vi "Complete Call on Error.vi"(8 "error in":errorcluster, 11 "gRPC ID in":T1) -> (0 "error out":errorcluster)   [LabVIEW 2021, in "NI Measurement Plug-In SDK.lvlib" / "IMeasurement Service.lvclass"]
uses:
  IMeasurement Service.lvclass
  <vilib>/gRPC/LabVIEW gRPC Library/Shared/grpcId.ctl
  <vilib>/gRPC/LabVIEW gRPC Library/Server API/typeDefs/gRPC Status Code.ctl
  <vilib>/Utility/error.llb/DialogType.ctl
  <vilib>/gRPC/LabVIEW gRPC Library/grpc-lvsupport-release.lvlib
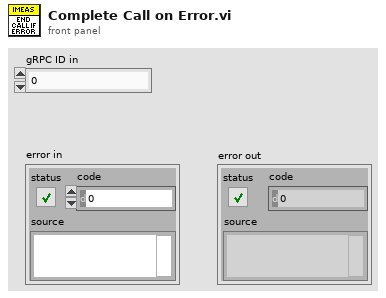
[diagram p1: front panel]
types:
  T1 = typedef "grpc-lvsupport-release.lvlib/grpcId.ctl" = u64
  T2 = typedef "grpc-lvsupport-release.lvlib/gRPC Status Code.ctl" = enum16{"OK", "CANCELLED", "UNKNOWN", "INVALID_ARGUMENT", "DEADLINE_EXCEEDED", "NOT_FOUND", "ALREADY_EXISTS", "PERMISSION_DENIED", "RESOURCE_EXHAUSTED", "FAILED_PRECONDITION", "ABORTED", "OUT_OF_RANGE", "UNIMPLEMENTED", "INTERNAL", "UNAVAILABLE", "DATA_LOSS", "UNAUTHENTICATED"}
  T3 = typedef "DialogType.ctl" = u16
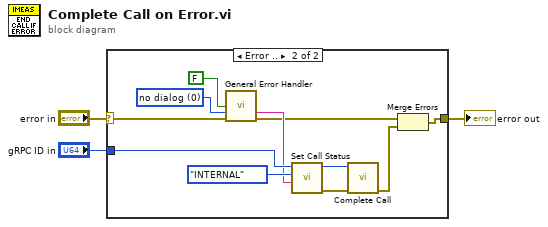
[diagram p0: block diagram]
diagram:
  n1 = case shown="Error .." "error in" {
    selector: "error in" -> [w4 w13]
    tunnel: [w4 w5] -> w1
    tunnel: "gRPC ID in" -> [_ w14]
    frame No Error {
      # "no error: pass through"
    }
    frame Error {
      w11 = T3 0 items=["no dialog", "OK message", "continue or stop message", "OK message + warnings", "continue/stop + warnings"] ("type of dialog (OK msg:1)")
      # "Report any errors over the grpc response."
      n2 = call <vilib>:"General Error Handler.vi"("search ni.com link visible?(T)"=FALSE, "type of dialog (OK msg:1)"=w11, "error in (no error)"=w13) -> ("message"=w12:string, "error out"=w6:errorcluster)  [unwired: 8 in, 3 out]
      n3 = call <vilib>:"Set Call Status.vi"("Details"=w12, "Status Code"=gRPC_Status_Code."INTERNAL", "gRPCid in"=w14) -> ("error out"=w9:errorcluster, "gRPCid out"=w8:T1)  [unwired: 7 in]
      n4 = call <vilib>:"Complete Call.vi"("gRPCid"=w8, "error in"=w9) -> ("error out"=w7:errorcluster)  [unwired: 8 in]
      n5 = Merge Errors(w6, w7) -> (w5:errorcluster)
    }
  }
  "error out" <- w1
